vi "AlliGator Get All Ancillary Window Paths.vi"(8 "Error In":errorcluster) -> (0 "Error Out":errorcluster, 3 "AlliGator Window Paths":path[](array[path]))   [LabVIEW 2021, in "AlliGator GUI.lvlib"]
doc: "Returns the paths of all AlliGator windows (except those not close when quitting).\nThis is used when quitting AlliGator."
uses:
  AlliGator GUI.lvlib
  AlliGator Windows List.ctl
  <userlib>/_OpenG.lib/array/array.llb/Filter 1D Array (U16)__ogtk.vi
  <userlib>/_OpenG.lib/array/array.llb/openg_array.lvlib
panel:
  # "see the AlliGator License on the block diagram (Ctrl+E or Window:Show Block Diagram)"
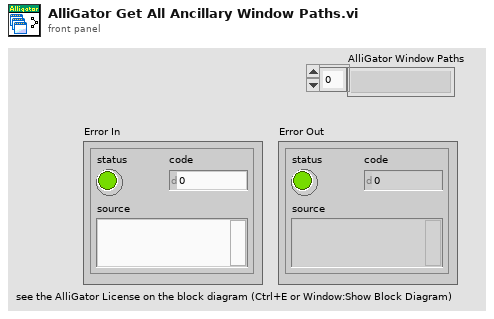
[diagram p1: front panel]
types:
  T1 = typedef "AlliGator GUI.lvlib/AlliGator Windows List.ctl" = enum16{"AlliGator Window", "Settings Window", "Notebook Window", "Dataset Information Window", "Source Image ROI Manager Window", "Phasor Plot ROI Manager Window", "Phasor Harmonic Manager Window", "Histogram Window", "Image Profile Window", "Local Decay Window", "About Window", "Batch Conversion Window", "Shot Noise Influence on Average Lifetime", "Fit Method Benchmark", "AlliGator Alias Definition"}
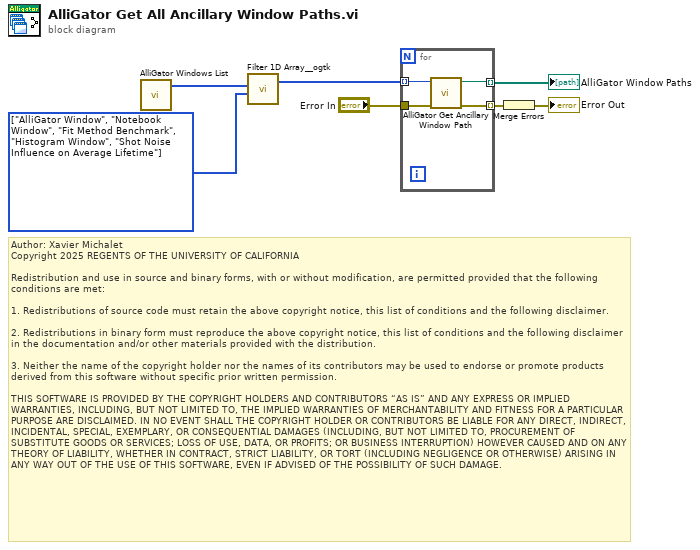
[diagram p0: block diagram]
diagram:
  w2 = T1[] [enum."AlliGator Window", enum."Notebook Window", enum."Fit Method Benchmark", enum."Histogram Window", enum."Shot Noise Influence on Average Lifetime"] items=["AlliGator Window", "Settings Window", "Notebook Window", "Dataset Information Window", "Source Image ROI Manager Window", "Phasor Plot ROI Manager Window", "Phasor Harmonic Manager Window", "Histogram Window", "Image Profile Window", "Local Decay Window", "About Window", "Batch Conversion Window", "Shot Noise Influence on Average Lifetime", "Fit Method Benchmark", "AlliGator Alias Definition"] ("AlliGator Windows List")
  # "Author: Xavier Michalet\nCopyright 2025 REGENTS OF THE UNIVERSITY OF CALIFORNIA\n\nRedistribution and use in source and binary forms, with or without modification, are permitted provided that the following conditions are met:\n\n1. Redistributions of source code must retain the above copyright notice, this list of conditions and the following disclaimer.\n\n2. Redistributions in binary form must reproduce the above copyright notice, this list of conditions and the following disclaimer in the documentation and/or other materials provided with the distribution.\n\n3. Neither the name of the copyright holder nor the names of its contributors may be used to endorse or promote products derived from this software without specific prior written permission.\n\nTHIS SOFTWARE IS PROVIDED BY THE COPYRIGHT HOLDERS AND CONTRIBUTORS “AS IS” AND ANY EXPRESS OR IMPLIED WARRANTIES, INCLUDING, BUT NOT LIMITED TO, THE IMPLIED WARRANTIES OF MERCHANTABILITY AND FITNESS FOR A PARTICULAR PURPOSE ARE DISCLAIMED. IN NO EVENT SHALL THE COPYRIGHT HOLDER OR CONTRIBUTORS BE LIABLE FOR ANY DIRECT, INDIRECT, INCIDENTAL, SPECIAL, EXEMPLARY, OR CONSEQUENTIAL DAMAGES (INCLUDING, BUT NOT LIMITED TO, PROCUREMENT OF SUBSTITUTE GOODS OR SERVICES; LOSS OF USE, DATA, OR PROFITS; OR BUSINESS INTERRUPTION) HOWEVER CAUSED AND ON ANY THEORY OF LIABILITY, WHETHER IN CONTRACT, STRICT LIABILITY, OR TORT (INCLUDING NEGLIGENCE OR OTHERWISE) ARISING IN ANY WAY OUT OF THE USE OF THIS SOFTWARE, EVEN IF ADVISED OF THE POSSIBILITY OF SUCH DAMAGE."
  n1 = call "AlliGator Windows List.vi"() -> ("AlliGator Windows List"=w3:T1[])  [unwired: 11 in]
  n2 = call-poly <userlib>:"Filter 1D Array__ogtk.vi"("items to filter"=w2, "array"=w3) -> ("filtered array"=w1:u16[])  [unwired: 4 in, 1 out]
  n3 = for {
    tunnel: w1 -> [w11] mode=indexing
    tunnel: [w10] -> w7 mode=indexing
    tunnel: [w9] -> w6 mode=indexing
    tunnel: "Error In" -> [w8]
    n4 = call "AlliGator Get Ancillary Window Path.vi"("Error In"=w8, "AlliGator Window"=w11) -> ("Error Out"=w9:errorcluster, "VI Path"=w10:path)  [unwired: 8 in]
  }
  "AlliGator Window Paths" <- w7
  n5 = Merge Errors(w6) -> (→"Error Out":errorcluster)
